vi "Get Traces.vi"(4 "Filter?":bool, 6 "max points per trace (all)":i32=-1, 7 "time_bucket":T1(ring), 8 "error in (no error)":errorcluster, 9 "time interval":T3, 10 "Trace names":string[](array[string]), 11 "Database Viewer.lvclass":refnum<class "Database Viewer.lvclass">) -> (0 "error out":errorcluster, 1 "SQL":string, 2 "Traces Out":T2(array[cluster]), 3 "Database Viewer.lvclass":refnum<class "Database Viewer.lvclass">)   [LabVIEW 2019, in "Database Viewer.lvclass"]
uses:
  Database Viewer.lvclass
  Database Viewer.lvclass/Database Viewer.ctl
  <userlib>/LevyLab/LV-Data/LV-Data.PG/LV-Data.PGSQL.lvclass
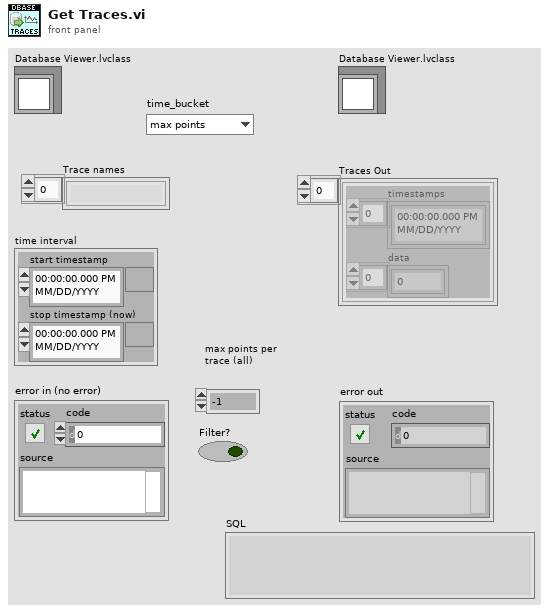
[diagram p1: front panel]
types:
  T1 = enum16{"max points", "1 second", "5 seconds", "10 seconds", "30 seconds", "1 minute", "5 minutes", "10 minutes", "30 minutes", "1 hour", "5 hours", "10 hours", "30 hours"}
  T2 = cluster{"timestamps":timestamp[], "data":dbl[]}[]
  T3 = cluster{"start timestamp":timestamp, "stop timestamp (now)":timestamp}
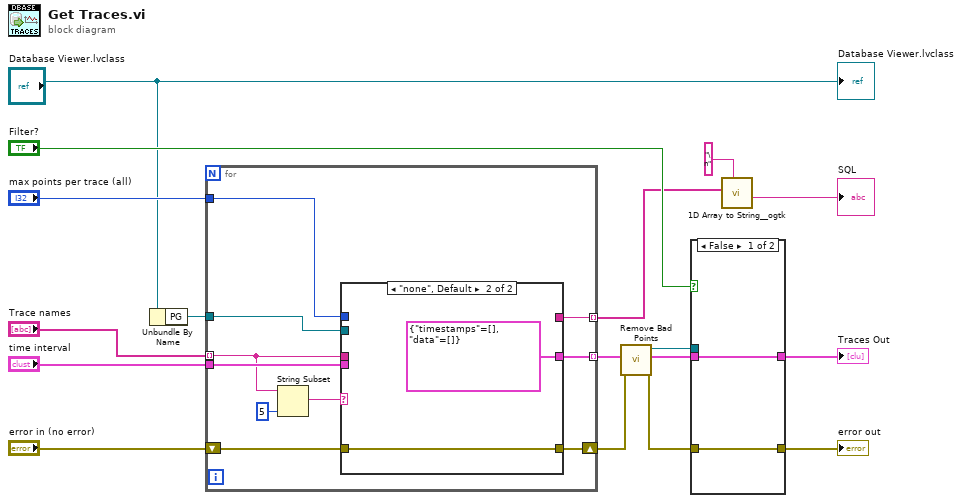
[diagram p0: block diagram]
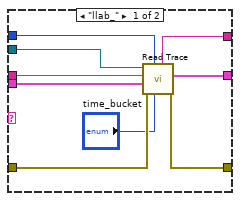
[diagram p2: hidden frame]
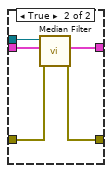
[diagram p3: hidden frame]
diagram:
  n1 = Unbundle By Name("Database Viewer.lvclass") -> ("PG"=w10:refnum<class "LV-Data.PGSQL.lvclass">)
  n2 = for {
    tunnel: "Trace names" -> [w19] mode=indexing
    tunnel: [w26] -> w3 mode=indexing
    tunnel: "time interval" -> [w27]
    tunnel: "max points per trace (all)" -> [w25]
    tunnel: w10 -> [w23]
    shift-right: [w20] -> w12
    shift-left: "error in (no error)" -> [w21]
    tunnel: [w18] -> w7 mode=indexing
    n3 = String Subset(string=w19, length (rest)=5 ("length (rest)")) -> (substring=w22:string)  [unwired: 1 in]
    n4 = case shown="\"none\", Default" w22 {
      tunnel: w27 -> [w34 _]
      tunnel: [w36 cluster{"timestamps":timestamp[], "data":dbl[]} {"timestamps"=[], "data"=[]} ("Trace")] -> w26
      tunnel: w25 -> [w33 _]
      tunnel: w19 -> [w30 _]
      tunnel: w23 -> [w35 _]
      tunnel: w21 -> [w32 w37]
      tunnel: [w31 w37] -> w20
      tunnel: [w29 _] -> w18
      frame "llab_" {
        n5 = call <userlib>:"Read Trace.vi"("time_bucket"="time_bucket", "max points (-1 = all)"=w33, "error in (no error)"=w32, "time interval"=w34, "PG path"=w30, "Data.PGQL in"=w35) -> ("error out"=w31:errorcluster, "Trace"=w36:cluster{timestamp[], dbl[]}, "SQL string"=w29:string)  [unwired: 1 in, 2 out]
      }
      frame "none", Default {
      }
    }
  }
  n6 = call "Remove Bad Points.vi"("error in (no error)"=w12, "Database Trace In"=w3) -> ("error out"=w9:errorcluster, "Database Trace Out"=w2:T2, "Database Viewer out"=w1:refnum<class "Database Viewer.lvclass">)  [unwired: 7 in]
  n7 = case shown="False" "Filter?" {
    tunnel: w1 -> [_ w43]
    tunnel: [w39 w41] -> w4
    tunnel: w9 -> [w40 w45]
    tunnel: [w40 w44] -> w11
    tunnel: w2 -> [w39 w42]
    frame False {
    }
    frame True {
      n8 = call "Median Filter.vi"("error in (no error)"=w45, "Database Trace"=w42, "Database Viewer"=w43) -> ("error out"=w44:errorcluster, "Database Trace out"=w41:T2)  [unwired: 6 in, 1 out]
    }
  }
  "Traces Out" <- w4
  "error out" <- w11
  n9 = call <userlib>:"1D Array to String__ogtk.vi"("delimiter (Tab)"="\n", "Array of Strings"=w7) -> ("delimited string"=→"SQL":string)  [unwired: 9 in]
  "Database Viewer.lvclass" <- "Database Viewer.lvclass"
